vi "GetFormattedStringBounds.vi"(0 "reference":refnum<class "MultiLineString.lvclass">, 1 "graphics":refnum<class "Graphics.lvclass">, 5 "error in (no error)":errorcluster, 6 "TargetBounds(IgnoreIfZero)":T1 {"height" format="%.2f"; "width" format="%.2f"; "y" format="%.2f"; "x" format="%.2f"}) -> (14 "reference out":refnum<class "MultiLineString.lvclass">, 15 "bounds":T1 {"height" format="%.2f"; "width" format="%.2f"; "y" format="%.2f"; "x" format="%.2f"}, 19 "error out":errorcluster)   [LabVIEW 2014, in "MultiLineString.lvclass"]
doc: "public Rectangle2D getBounds(Graphics2D g2)"
uses:
  <resource>/Framework/Providers/Open_GDS/UML/MultiLineString_class/MultiLineString.lvclass
  <resource>/Framework/Providers/Open_GDS/UML/General/Rectangle/Rectangle Rectangle2D.ctl
  <resource>/Framework/Providers/Open_GDS/UML/Graphics_class/Graphics.lvclass
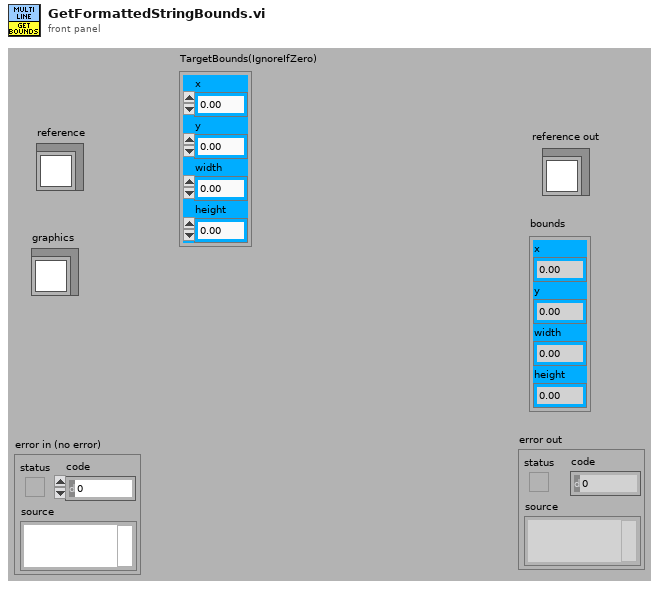
[diagram p1: front panel]
types:
  T1 = typedef "Rectangle Rectangle2D.ctl" = cluster{"x":dbl, "y":dbl, "width":dbl, "height":dbl}
  T2 = typedef "MultiLineString.lvclass/ObjectAttributes.ctl" = cluster{"GAP":i32, "text":string, "justification":T3, "size":T4, "underlined":bool}
  T3 = typedef "MultiLineString.lvclass/JustificationType.ctl" = enum16{"LEFT", "CENTER", "RIGHT"}
  T4 = typedef "MultiLineString.lvclass/SizeType.ctl" = enum16{"LARGE", "NORMAL", "SMALL"}
  T5 = typedef "Graphics.lvclass/FontType.ctl" = cluster{"Font Name:":string, "Size":i16, "Strikeout?":bool, "Italic?":bool, "Underline?":bool, "Outline?":bool, "Shadow?":bool, "Bold?":bool}
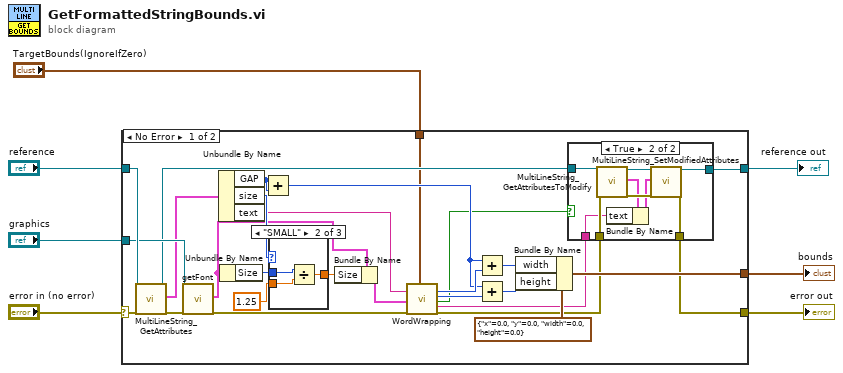
[diagram p0: block diagram]
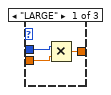
[diagram p3: hidden frame]
diagram:
  n1 = case shown="No Error" "error in (no error)" {
    selector: "error in (no error)" -> [w32 w54]
    tunnel: "reference" -> [w35 w55]
    tunnel: [w12 w54] -> w6
    tunnel: [w11 w55] -> w5
    tunnel: [w34 _] -> w3
    tunnel: "graphics" -> [w33 _]
    tunnel: "TargetBounds(IgnoreIfZero)" -> [w8 _]
    frame No Error {
      n2 = call <resource>:"MultiLineString_GetAttributes.vi"("reference in"=w35, "error in (no error)"=w32) -> ("reference out"=w14:refnum<class "MultiLineString.lvclass">, "Attributes"=w31:T2, "error out"=w18:errorcluster)  [unwired: 15 out]
      n3 = call <resource>:"getFont.vi"("reference"=w33, "error in (no error)"=w18) -> ("font"=w27:T5, "error out"=w16:errorcluster)  [unwired: 16 out]
      n4 = Unbundle By Name(w31) -> ("GAP"=w25:i32, "size"=w28:T4, "text"=w23:string)
      n5 = Unbundle By Name(w27) -> ("Size"=w30:i16)
      n6 = Add(x=w25, y=w25) -> (x+y=w21:i32)
      n7 = case shown="\"SMALL\"" w28 {
        tunnel: w30 -> [w49 w51 w53]
        tunnel: 1.25 ("y") -> [w48 w52 _]
        tunnel: [w47 w50 w53] -> w26
        frame "LARGE" {
          n8 = Multiply(x=w49, y=w48) -> (x*y=w47:dbl)
        }
        frame "SMALL" {
          n9 = Divide(x=w51, y=w52) -> (x/y=w50:dbl)
        }
        frame "NORMAL", Default {
        }
      }
      n10 = Bundle By Name(cluster=w27, "Size"=w26) -> (w17:T5)
      n11 = call <resource>:"WordWrapping.vi"("FormattedMultiLineStringIn"=w23, "Font"=w17, "error in (no error)"=w16, "TargetBounds(IgnoreIfZero)"=w8) -> ("Width"=w22:i16, "Height"=w20:i16, "StringWrapped"=w9:bool, "WrappedFormattedMultiLineStringOut"=w10:string, "error out"=w13:errorcluster)  [unwired: 11 in]
      n12 = Add(x=w21, y=w22) -> (x+y=w24:i32)
      n13 = Add(x=w21, y=w20) -> (x+y=w19:i32)
      n14 = Bundle By Name(cluster=T1 {"x"=0.0, "y"=0.0, "width"=0.0, "height"=0.0} ("bounds"), "width"=w24, "height"=w19) -> (w34:T1)
      n15 = case shown="True" w9 {
        tunnel: w14 -> [w37 w44]
        tunnel: w13 -> [w36 w43]
        tunnel: [w36 w42] -> w12
        tunnel: [w37 w41] -> w11
        tunnel: w10 -> [_ w38]
        frame False {
        }
        frame True {
          n16 = call <resource>:"MultiLineString_GetAttributesToModify.vi"("reference in"=w44, "error in (no error)"=w43) -> ("reference out"=w45:refnum<class "MultiLineString.lvclass">, "Attributes"=w40:T2, "error out"=w46:errorcluster)  [unwired: 14 in, 1 out]
          n17 = Bundle By Name(cluster=w40, "text"=w38) -> (w39:T2)
          n18 = call <resource>:"MultiLineString_SetModifiedAttributes.vi"("reference in"=w45, "Attributes"=w39, "error in (no error)"=w46) -> ("reference out"=w41:refnum<class "MultiLineString.lvclass">, "error out"=w42:errorcluster)  [unwired: 15 in]
        }
      }
    }
    frame Error {
    }
  }
  "reference out" <- w5
  "error out" <- w6
  "bounds" <- w3
